vi "FilterOutProbes.vi"(0 "Exists at index":i32, 2 "Item Name":string) -> (7 "Include?":bool)   [LabVIEW 2013]
doc: "Custom probes are included in the App.AllVIs list. These entries, since they do not have a filename extension, will cause errors in the \"Compare Two Paths\" VI when it is called downstream. This VI removes the names of custom probes from the list, hence suppressing the errors."
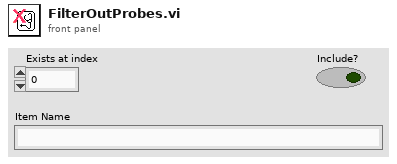
[diagram p1: front panel]
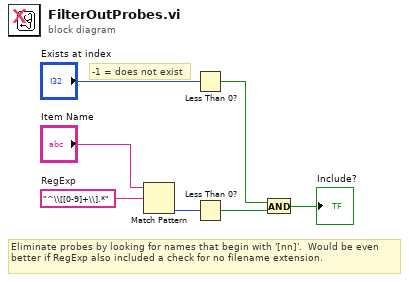
[diagram p0: block diagram]
diagram:
  w4 = "^\\[[0-9]+\\].*"  # RegExp
  # "-1 = does not exist"
  # "Eliminate probes by looking for names that begin with '[nn]'.  Would be even better if RegExp also included a check for no filename extension."
  n1 = Match Pattern(string="Item Name", regular expression=w4) -> (offset past match=w5:i32)  [unwired: 1 in, 3 out]
  n2 = Less Than 0?(x="Exists at index") -> (x < 0?=w1:bool)
  n3 = Less Than 0?(x=w5) -> (x < 0?=w6:bool)
  n4 = And(x=w1, y=w6) -> (x .and. y?=→"Include?":bool)
